vi "InternalStacking.vi"() -> ()   [LabVIEW 2014]
uses:
  InternalStacking.ctl
panel:
  in  "State of Elevator":T1
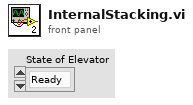
[diagram p1: front panel]
types:
  T1 = typedef "InternalStacking.ctl" = enum16{"Ready", "Extend Plate", "Lift Tote", "Wait For Seated Tote", "Release Tote", "Reset To Bottom Limit "}
  T2 = typedef "WPI_JoystickDevRef.ctl" = cluster{"Device":T3}
  T3 = typedef "WPI_JoystickDeviceEnum.ctl" = enum16{"USB 0", "USB 1", "USB 2", "USB 3", "USB 4", "USB 5"}
  T4 = cluster{"Buttons[0]":bool, "Buttons[1]":bool, "Buttons[2]":bool, "Buttons[3]":bool, "Buttons[4]":bool, "Buttons[5]":bool, "Buttons[6]":bool, "Buttons[7]":bool, "Buttons[8]":bool}
  T5 = typedef "WPI_ServoDeviceRef.ctl" = cluster{"DeviceStatus":errorcluster, "Controller":T6, "PWM Channel":T7, "DeadBand":T8}
  T6 = typedef "FPGA_TypedefDigitalModule.ctl" = enum16{"Controller 1"}
  T7 = typedef "FPGA_DIOPWMChannel.ctl" = enum8{"PWM 0", "PWM 1", "PWM 2", "PWM 3", "PWM 4", "PWM 5", "PWM 6", "PWM 7", "PWM 8", "PWM 9", "PWM MXP 0", "PWM MXP 1", "PWM MXP 2", "PWM MXP 3", "PWM MXP 4", "PWM MXP 5", "PWM MXP 6", "PWM MXP 7", "PWM MXP 8", "PWM MXP 9", "Invalid"}
  T8 = typedef "WPI_PWMDeadband.ctl" = cluster{"Name":string, "maxPositivePwm":i32, "minPositivePwm":i32, "centerPwm":i32, "maxNegativePwm":i32, "minNegativePwm":i32, "angularRange":u16}
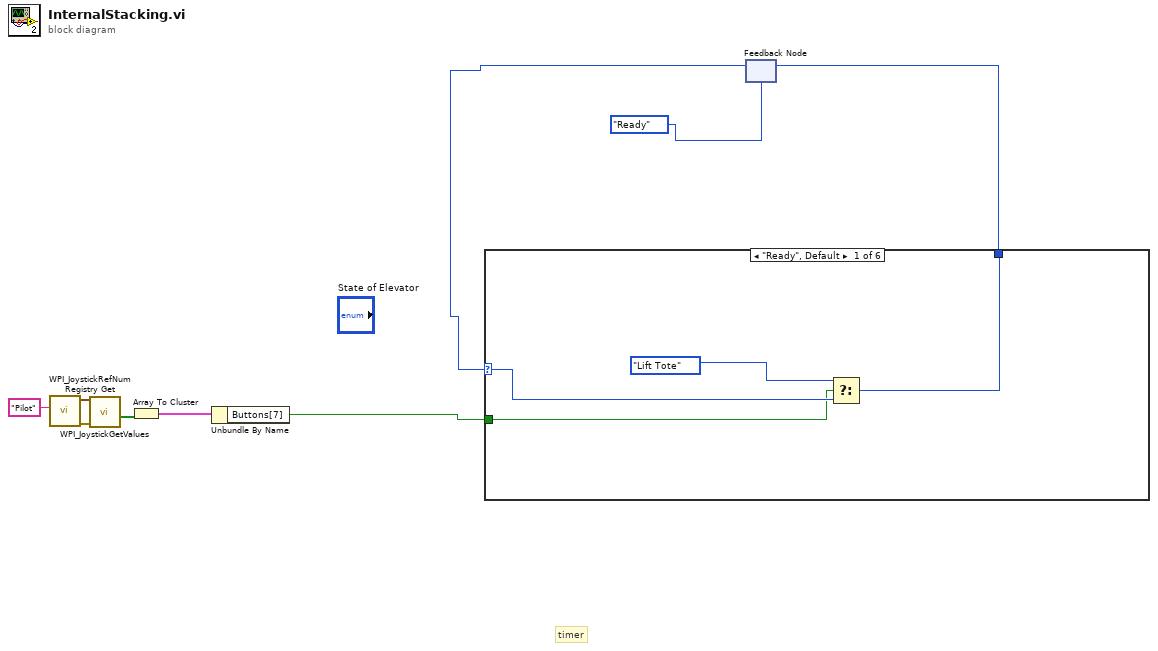
[diagram p0: block diagram]
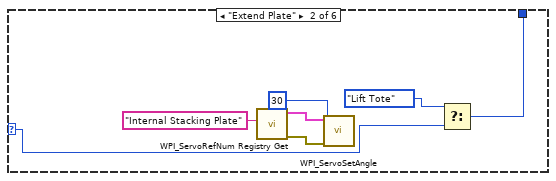
[diagram p2: hidden frame]
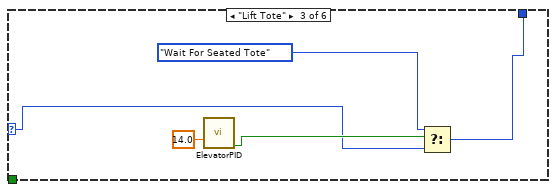
[diagram p3: hidden frame]
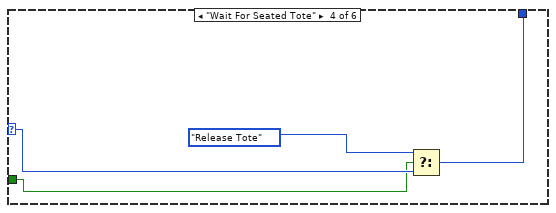
[diagram p4: hidden frame]
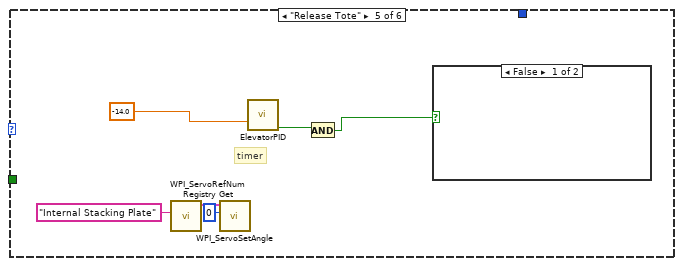
[diagram p5: hidden frame]
diagram:
  # "timer"
  n1 = call <vilib>:"WPI_JoystickRefNum Registry Get.vi"("refnum name"="Pilot") -> ("error out"=w8:errorcluster, "JoystickDevRef"=w7:T2)  [unwired: 9 in]
  n2 = call <vilib>:"WPI_JoystickGetValues.vi"("error in (no error)"=w8, "JoystickDevRef"=w7) -> ("Buttons"=w6:bool[])  [unwired: 5 in, 4 out]
  n3 = Array To Cluster(array=w6) -> (cluster=w5:T4)
  n4 = Unbundle By Name(w5) -> ("Buttons[7]"=w2:bool)
  n5 = feedback #1(InternalStacking."Ready" ("State of Elevator")) -> (w3:T1)
  n6 = case shown="\"Ready\", Default" w3 {
    selector: w3 -> [w12 w15 w22 w28 _ _]
    tunnel: w2 -> [w11 _ _ w27 _ _]
    tunnel: [w10 w14 w21 w26 _ _] -> w1
    frame "Ready", Default {
      n7 = Select(t=InternalStacking."Lift Tote" ("State of Elevator"), s=w11, f=w12) -> (s? t:f=w10:T1)
    }
    frame "Extend Plate" {
      n8 = call <vilib>:"WPI_ServoRefNum Registry Get.vi"("refnum name"="Internal Stacking Plate") -> ("error out"=w19:errorcluster, "ServoDeviceRef"=w18:T5)  [unwired: 9 in]
      n9 = call <vilib>:"WPI_ServoSetAngle.vi"("error in (no error)"=w19, "Angle"=30, "ServoDeviceRef"=w18) -> ()  [unwired: 7 in, 2 out]
      n10 = Select(t=InternalStacking."Lift Tote" ("State of Elevator"), f=w15) -> (s? t:f=w14:T1)  [unwired: 1 in]
    }
    frame "Lift Tote" {
      n11 = call "ElevatorPID.vi"("Elevator Setpoint"=14.0) -> ("At Setpoint"=w24:bool)  [unwired: 14 in]
      n12 = Select(t=InternalStacking."Wait For Seated Tote" ("State of Elevator"), s=w24, f=w22) -> (s? t:f=w21:T1)
    }
    frame "Wait For Seated Tote" {
      n13 = Select(t=InternalStacking."Release Tote" ("State of Elevator"), s=w27, f=w28) -> (s? t:f=w26:T1)
    }
    frame "Release Tote" {
      # "timer"
      n14 = call <vilib>:"WPI_ServoRefNum Registry Get.vi"("refnum name"="Internal Stacking Plate") -> ("ServoDeviceRef"=w32:T5)  [unwired: 9 in, 1 out]
      n15 = call <vilib>:"WPI_ServoSetAngle.vi"("Angle"=0, "ServoDeviceRef"=w32) -> ()  [unwired: 8 in, 2 out]
      n16 = call "ElevatorPID.vi"("Elevator Setpoint"=-14.0) -> ("At Setpoint"=w34:bool)  [unwired: 14 in]
      n17 = And(x=w34) -> (x .and. y?=w30:bool)  [unwired: 1 in]
      n18 = case shown="False" w30 {
        frame False {
        }
        frame True {
        }
      }
    }
    frame "Reset To Bottom Limit " {
    }
  }
  n19 = feedback-in #1(w1) -> ()
